vi "FPGA AIT 429 RT Driver VI.vi"(7 "Operation":T1, 11 "Device Reference in":T2 format="%.0x") -> (0 "Error Code":i32)   [LabVIEW 2012]
uses:
  <vilib>/NI Veristand/Custom Device API/Custom Device Item Ref.ctl
  <vilib>/NI Veristand/Custom Device API/Hardware Interface Driver VI Operation.ctl
  <vilib>/NI Veristand/Custom Device API/Custom Device Channel Type.ctl
  <vilib>/NI Veristand/Custom Device API/Data Reference.ctl
  SEA 9811 FPGA driver/RT/Typdefs/SEA9811_RT_data_cluster.ctl
  SEA 9811 FPGA driver/RT/Typdefs/FPGA ref.ctl
  SEA 9811 FPGA driver/RT/Typdefs/SEA9811_RT_conf_cluster.ctl
  <vilib>/userdefined/High Color/nirio_resource_hc.ctl
  SEA 9811 FPGA driver/FPGA/SEA-9811_ReceiverAndTransmitter/SubVIs/SEA-9811_ReceiverAndTransmitter_RCR.ctl
  SEA 9811 FPGA driver/FPGA/SEA-9811_ReceiverAndTransmitter/SubVIs/SEA-9811_ReceiverAndTransmitter_TCR.ctl
  <vilib>/NI Veristand/Custom Device API/Data Access Type.ctl
  <vilib>/NI Veristand/Custom Device API/Get Item Property (String).vi
  SEA 9811/Source/Shared/Constants.vi
  <vilib>/NI Veristand/Custom Device API/Global Data Refs.vi
  <vilib>/NI Veristand/Custom Device API/Custom Device API.lvlib
  SEA 9811/Source/Shared/SEA 9811 Shared.lvlib
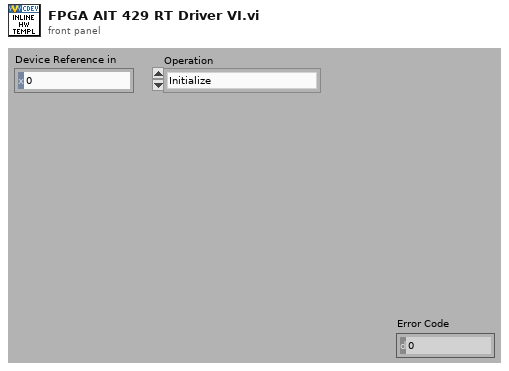
[diagram p1: front panel]
types:
  T1 = typedef "Custom Device API.lvlib/Hardware Interface Driver VI Operation.ctl" = enum16{"Initialize", "Start", "Read Data from HW", "Write Data to HW", "Close"}
  T2 = typedef "Custom Device API.lvlib/Custom Device Item Ref.ctl" = u64
  T3 = typedef "Custom Device API.lvlib/Data Reference.ctl" = i32
  T4 = typedef "SEA9811_RT_data_cluster.ctl" = cluster{"FPGA VI Reference":T5, "Incoming channels":dbl[], "words_timestamps":dbl[]}
  T5 = typedef "FPGA ref.ctl" = refnum<k20>
  T6 = cluster{"Input Values":dbl[], "Input Refs":T3[], "Output Values":dbl[], "Output Refs":T3[], "SEA9811_RT_data out":T4, "Device Error":errorcluster}
  T7 = typedef "SEA9811_RT_conf_cluster.ctl" = cluster{"FPGA resource name":T8, "Rx ch conf (0..7)":cluster{"Rx Channel Number (0..7)":u8, "Rx Label Filter":cluster{"Label 00":u8, "Label 01":u8, "Label 02":u8, "Label 03":u8, "Label 04":u8, "Label 05":u8, "Label 06":u8, "Label 07":u8, "Label 08":u8, "Label 09":u8, "Label 10":u8, "Label 11":u8, "Label 12":u8, "Label 13":u8, "Label 14":u8, "Label 15":u8}, "Receiver Control Register (RCR)":T9}[], "Transmitter Control Register (TCR)":T10}
  T8 = typedef "nirio_resource_hc.ctl" = tag
  T9 = typedef "SEA-9811_ReceiverAndTransmitter_RCR.ctl" = cluster{"RCR0: Data rate = ARINC 429 High-Speed (0) or Low-Speed (1)":bool, "RCR1: not used":bool, "RCR2: Label recognition for this channel enabled (1) or disabled (0)":bool, "RCR3: Receiver channel disabled (1) or enabled (0)":bool, "RCR4: Odd parity check for this channel enabled (1) or disabled (0":bool, "RCR5: Receiver normal operation (1) or loopback mode (0)":bool, "RCR6: Receiver Decoder disabled (0) or enabled (1) -> ARINC bits 10 and 9 must match RCR7 and RCR8":bool, "RCR7: If receiver decoder is enabled (RCR6=1), the ARINC bit 10 must match this bit":bool, "RCR8: If receiver decoder is enabled (RCR6=1), the ARINC bit 9 must match this bit":bool, "RCR9: Label bit order for this channel non-reversed (1) or reversed (0)":bool, "RCR10: not used":bool, "RCR11: not used":bool, "RCR12: not used":bool, "RCR13: not used":bool, "RCR14: not used":bool, "RCR15: not used":bool}
  T10 = typedef "SEA-9811_ReceiverAndTransmitter_TCR.ctl" = cluster{"TCR0: not used":bool, "TCR1: not used":bool, "TCR2: not used":bool, "TCR3: Transmitter Parity Bit Enable: 32nd bit is parity (1) or data (0)":bool, "TCR4: not used":bool, "TCR5: not used":bool, "TCR6: not used":bool, "TCR7: not used":bool, "TCR8: not used":bool, "TCR9: Transmitter Parity Select: odd parity (0) or even parity (1)":bool, "TCR10: Transmitter Data Rate: ARINC 429 high-speed (0) or low-speed (1)":bool, "TCR11: ARINC Label Bit Order: label bit order reversed (0) or not reversed (1)":bool, "TCR12: Disable Line Driver: normal operation (0) or transmitter disabled (1)":bool, "TCR13: Tansmit whenever data is available in FIFO (1) or only start by instruction \"Enable Transmission\" (0)":bool, "TCR14: not used":bool, "TCR15: not used":bool}
  T11 = typedef "Custom Device API.lvlib/Custom Device Channel Type.ctl" = enum16{"Input", "Output"}
  T12 = typedef "Custom Device API.lvlib/Data Access Type.ctl" = enum16{"Read", "Write"}
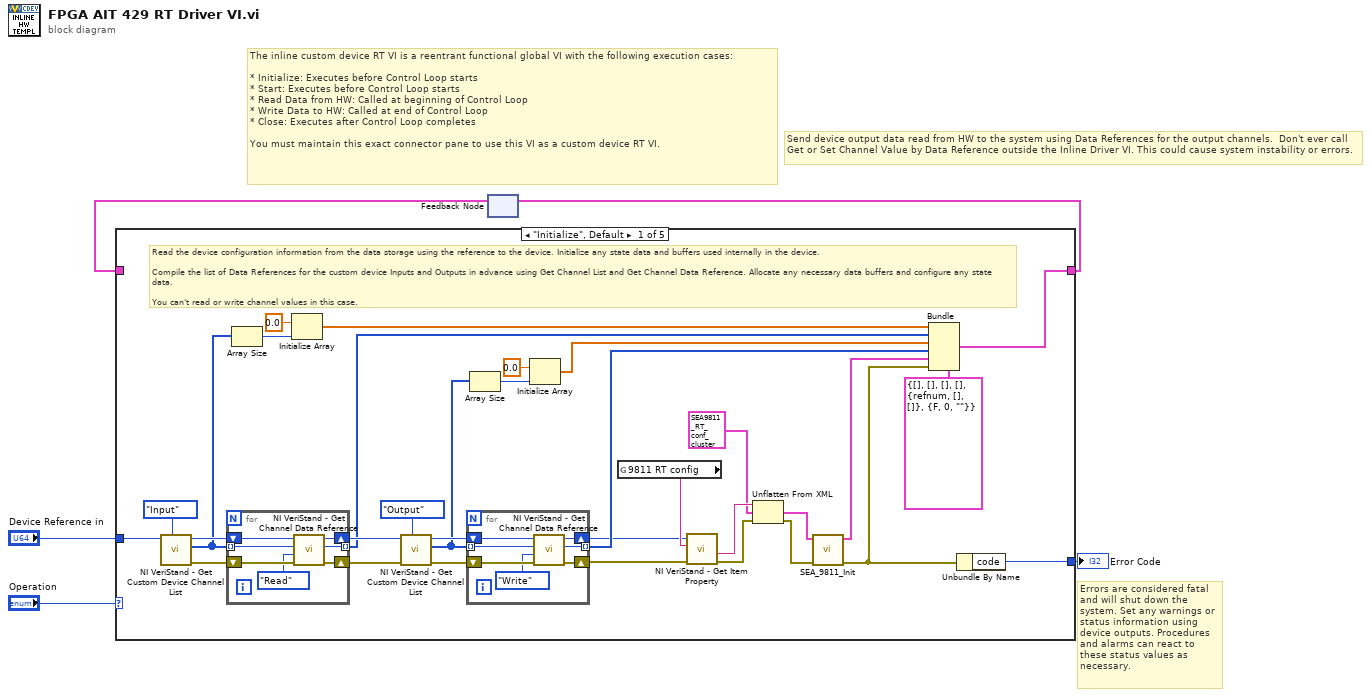
[diagram p0: block diagram]
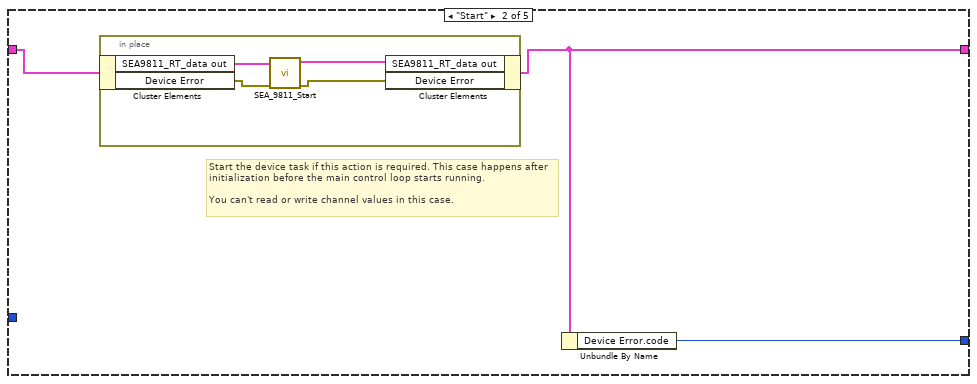
[diagram p2: hidden frame]
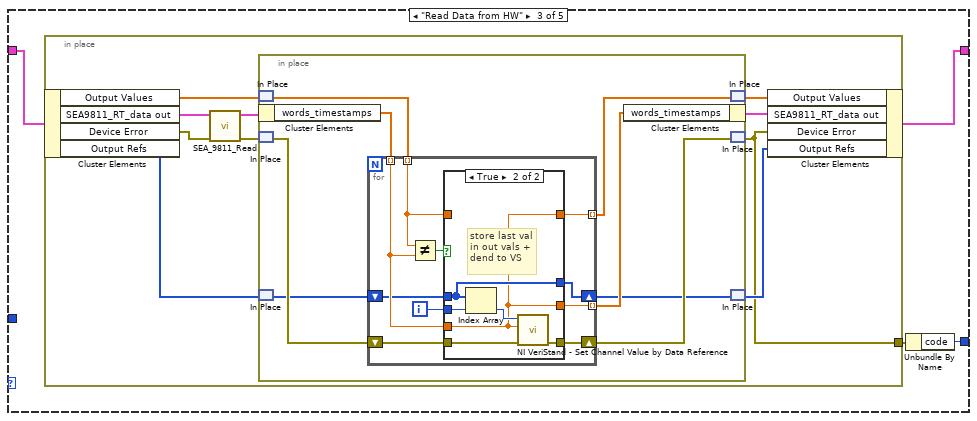
[diagram p3: hidden frame]
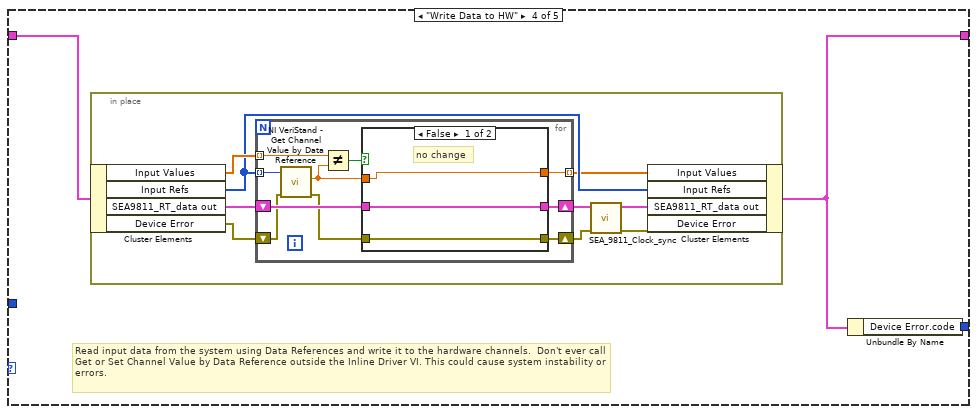
[diagram p5: hidden frame]
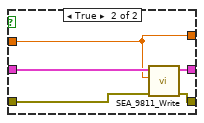
[diagram p6: hidden frame]
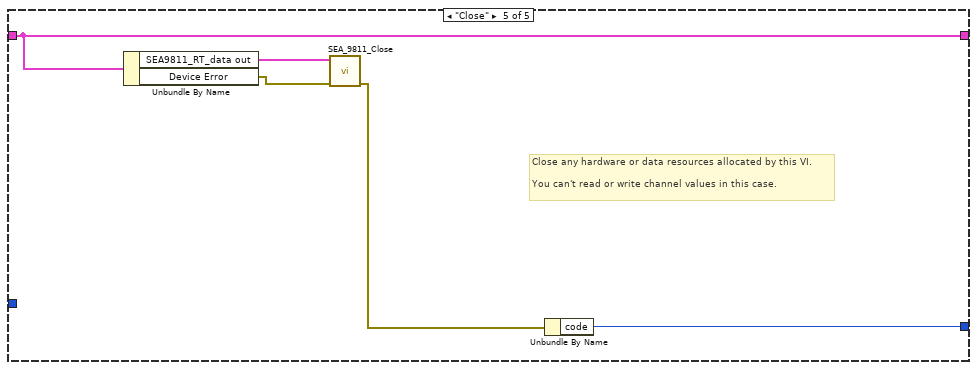
[diagram p7: hidden frame]
diagram:
  # "Send device output data read from HW to the system using Data References for the output channels.  Don't ever call Get or Set Channel Value by Data Reference outside the Inline Driver VI. This could cause system instability or errors."
  # "Errors are considered fatal and will shut down the system. Set any warnings or status information using device outputs. Procedures and alarms can react to these status values as necessary."
  # "The inline custom device RT VI is a reentrant functional global VI with the following execution cases:\n\n* Initialize: Executes before Control Loop starts\n* Start: Executes before Control Loop starts\n* Read Data from HW: Called at beginning of Control Loop\n* Write Data to HW: Called at end of Control Loop\n* Close: Executes after Control Loop completes\n\nYou must maintain this exact connector pane to use this VI as a custom device RT VI."
  n1 = feedback #1() -> (w3:T6)  [unwired: 1 out]
  n2 = case shown="\"Initialize\", Default" "Operation" {
    tunnel: [w32 w52 w60 w101 w131] -> w4
    tunnel: w3 -> [_ w53 w61 w102 w131]
    tunnel: "Device Reference in" -> [w33 _ _ _ _]
    tunnel: [w31 w54 w62 _ w134] -> w1
    frame "Initialize", Default {
      # "Read the device configuration information from the data storage using the reference to the device. Initialize any state data and buffers used internally in the device.\n\nCompile the list of Data References for the custom device Inputs and Outputs in advance using Get Channel List and Get Channel Data Reference. Allocate any necessary data buffers and configure any state data.\n\nYou can't read or write channel values in this case."
      n3 = call <vilib>:"NI VeriStand - Get Custom Device Channel List.vi"("Channel Type"=Custom_Device_Channel_Type."Input", "Device Ref in"=w33) -> ("error out"=w29:errorcluster, "Specified Channel Ref List"=w28:T2[], "Device Ref out"=w30:T2)  [unwired: 1 in, 6 out]
      n4 = for {
        shift-right: [w46] -> w24
        shift-left: w30 -> [w50]
        tunnel: w28 -> [w49] mode=indexing
        shift-right: [w47] -> w23
        shift-left: w29 -> [w51]
        tunnel: [w45] -> w22 mode=indexing
        n5 = call <vilib>:"NI VeriStand - Get Channel Data Reference.vi"("error in (no error)"=w51, "Access"=Data_Access_Type."Read", "Channel Ref in"=w49, "Device Ref in"=w50) -> ("error out"=w47:errorcluster, "Channel Data Reference"=w45:T3, "Device Ref out"=w46:T2)  [unwired: 5 out]
      }
      n6 = Array Size(array=w28) -> (size(s)=w36:i32)
      n7 = Initialize Array(0.0 ("element"), w36) -> (w37:dbl[])
      n8 = call <vilib>:"NI VeriStand - Get Custom Device Channel List.vi"("Channel Type"=Custom_Device_Channel_Type."Output", "error in (no error)"=w23, "Device Ref in"=w24) -> ("error out"=w27:errorcluster, "Specified Channel Ref List"=w19:T2[], "Device Ref out"=w26:T2)  [unwired: 6 out]
      n9 = for {
        tunnel: w19 -> [w42] mode=indexing
        shift-right: [w40] -> w8
        shift-left: w27 -> [w44]
        tunnel: [w39] -> w17 mode=indexing
        shift-right: [w38] -> w9
        shift-left: w26 -> [w43]
        n10 = call <vilib>:"NI VeriStand - Get Channel Data Reference.vi"("error in (no error)"=w44, "Access"=Data_Access_Type."Write", "Channel Ref in"=w42, "Device Ref in"=w43) -> ("error out"=w40:errorcluster, "Channel Data Reference"=w39:T3, "Device Ref out"=w38:T2)  [unwired: 5 out]
      }
      n11 = Array Size(array=w19) -> (size(s)=w20:i32)
      n12 = Initialize Array(0.0 ("element"), w20) -> (w18:dbl[])
      n13 = global read "Constants.vi" "9811 RT config"() -> (w13:string)
      n14 = call-poly <vilib>:"NI VeriStand - Get Item Property.vi"("error in (no error)"=w8, "Property Name"=w13, "Item Ref in"=w9) -> ("error out"=w11:errorcluster, "Value"=w12:string)  [unwired: 5 in, 2 out]
      n15 = Unflatten From XML(xml string=w12, type=T7 {"FPGA resource name"="RIO0", "Rx ch conf (0..7)"=[{"Rx Channel Number (0..7)"=0, "Rx Label Filter"={"Label 00"=0, "Label 01"=0, "Label 02"=0, "Label 03"=0, "Label 04"=0, "Label 05"=0, "Label 06"=0, "Label 07"=0, "Label 08"=0, "Label 09"=0, "Label 10"=0, "Label 11"=0, "Label 12"=0, "Label 13"=0, "Label 14"=0, "Label 15"=0}, "Receiver Control Register (RCR)"={"RCR0: Data rate = ARINC 429 High-Speed (0) or Low-Speed (1)"=FALSE, "RCR1: not used"=FALSE, "RCR2: Label recognition for this channel enabled (1) or disabled (0)"=FALSE, "RCR3: Receiver channel disabled (1) or enabled (0)"=FALSE, "RCR4: Odd parity check for this channel enabled (1) or disabled (0"=FALSE, "RCR5: Receiver normal operation (1) or loopback mode (0)"=TRUE, "RCR6: Receiver Decoder disabled (0) or enabled (1) -> ARINC bits 10 and 9 must match RCR7 and RCR8"=FALSE, "RCR7: If receiver decoder is enabled (RCR6=1), the ARINC bit 10 must match this bit"=FALSE, "RCR8: If receiver decoder is enabled (RCR6=1), the ARINC bit 9 must match this bit"=FALSE, "RCR9: Label bit order for this channel non-reversed (1) or reversed (0)"=FALSE, "RCR10: not used"=FALSE, "RCR11: not used"=FALSE, "RCR12: not used"=FALSE, "RCR13: not used"=FALSE, "RCR14: not used"=FALSE, "RCR15: not used"=FALSE}}], "Transmitter Control Register (TCR)"={"TCR0: not used"=FALSE, "TCR1: not used"=FALSE, "TCR2: not used"=FALSE, "TCR3: Transmitter Parity Bit Enable: 32nd bit is parity (1) or data (0)"=FALSE, "TCR4: not used"=FALSE, "TCR5: not used"=FALSE, "TCR6: not used"=FALSE, "TCR7: not used"=FALSE, "TCR8: not used"=FALSE, "TCR9: Transmitter Parity Select: odd parity (0) or even parity (1)"=FALSE, "TCR10: Transmitter Data Rate: ARINC 429 high-speed (0) or low-speed (1)"=FALSE, "TCR11: ARINC Label Bit Order: label bit order reversed (0) or not reversed (1)"=FALSE, "TCR12: Disable Line Driver: normal operation (0) or transmitter disabled (1)"=FALSE, "TCR13: Tansmit whenever data is available in FIFO (1) or only start by instruction \"Enable Transmission\" (0)"=TRUE, "TCR14: not used"=FALSE, "TCR15: not used"=FALSE}} ("SEA9811_conf_cluster 2"), error in (no error)=w11) -> (value=w6:T7, error out=w7:errorcluster)
      n16 = call "SEA_9811_Init.vi"("error in"=w7, "SEA9811_conf_cluster"=w6) -> ("error out"=w14:errorcluster, "SEA9811_RT_data out"=w15:T4)  [unwired: 8 in]
      n17 = Bundle(cluster=T6 {"Input Values"=[], "Input Refs"=[], "Output Values"=[], "Output Refs"=[], "SEA9811_RT_data out"={"FPGA VI Reference"=refnum, "Incoming channels"=[], "words_timestamps"=[]}, "Device Error"={"status"=FALSE, "code"=0, "source"=""}}, "Input Values"=w37, "Input Refs"=w22, "Output Values"=w18, "Output Refs"=w17, "SEA9811_RT_data out"=w15, "Device Error"=w14) -> (w32:T6)
      n18 = Unbundle By Name(w14) -> ("code"=w31:i32)
    }
    frame "Start" {
      # "Start the device task if this action is required. This case happens after initialization before the main control loop starts running.\n\nYou can't read or write channel values in this case."
      n19 = in-place {
        n20 = in-place-cluster #2(w53) -> ("SEA9811_RT_data out"=w58:T4, "Device Error"=w57:errorcluster)
        n21 = call "SEA_9811_Start.vi"("error in (no error)"=w57, "SEA9811_RT_data in"=w58) -> ("error out"=w55:errorcluster, "SEA9811_RT_data out"=w56:T4)  [unwired: 8 in]
        n22 = in-place-cluster #2("SEA9811_RT_data out"=w56, "Device Error"=w55) -> (w52:T6)
      }
      n23 = Unbundle By Name(w52) -> ("Device Error.code"=w54:i32)
    }
    frame "Read Data from HW" {
      n24 = in-place {
        in-place-border: [w64] -> w59
        n25 = in-place-cluster #3(w61) -> ("Output Values"=w69:dbl[], "SEA9811_RT_data out"=w71:T4, "Device Error"=w72:errorcluster, "Output Refs"=w67:T3[])
        n26 = call "SEA_9811_Read.vi"("error in (no error)"=w72, "SEA9811_RT_data in"=w71) -> ("error out"=w68:errorcluster, "SEA9811_RT_data out"=w70:T4)  [unwired: 6 in, 2 out]
        n27 = in-place {
          n28 = in-place-match #4(w69) -> (w79:dbl[])
          n29 = in-place-cluster #5(w70) -> ("words_timestamps"=w78:dbl[])
          n30 = in-place-match #6(w68) -> (w80:errorcluster)
          n31 = in-place-match #7(w67) -> (w77:T3[])
          n32 = for {
            tunnel: w79 -> [w84] mode=indexing
            tunnel: w78 -> [w89] mode=indexing
            shift-right: [w85] -> w74
            shift-left: w80 -> [w86]
            tunnel: [w83] -> w75 mode=indexing
            tunnel: [w82] -> w76 mode=indexing
            shift-right: [w81] -> w73
            shift-left: w77 -> [w88]
            i -> [w87]
            n33 = Not Equal?(x=w84, y=w89) -> (x != y?=w90:bool)
            n34 = case shown="True" w90 {
              tunnel: w89 -> [w91 w95]
              tunnel: w88 -> [w92 w96]
              tunnel: w87 -> [_ w100]
              tunnel: w86 -> [w94 w98]
              tunnel: [w94 w97] -> w85
              tunnel: w84 -> [w93 _]
              tunnel: [w93 w95] -> w83
              tunnel: [w91 w95] -> w82
              tunnel: [w92 w96] -> w81
              frame False {
              }
              frame True {
                # "store last val\nin out vals +\ndend to VS"
                n35 = Index Array(array=w96, index=w100) -> (element=w99:T3)
                n36 = call <vilib>:"NI VeriStand - Set Channel Value by Data Reference.vi"("error in (no error)"=w98, "Value"=w95, "Data Reference in"=w99) -> ("error out"=w97:errorcluster)  [unwired: 8 out]
              }
            }
          }
          n37 = in-place-cluster #5("words_timestamps"=w76) -> (w63:T4)
          n38 = in-place-match #4(w75) -> (w66:dbl[])
          n39 = in-place-match #6(w74) -> (w64:errorcluster)
          n40 = in-place-match #7(w73) -> (w65:T3[])
        }
        n41 = in-place-cluster #3("Output Values"=w66, "SEA9811_RT_data out"=w63, "Device Error"=w64, "Output Refs"=w65) -> (w60:T6)
      }
      n42 = Unbundle By Name(w59) -> ("code"=w62:i32)
    }
    frame "Write Data to HW" {
      # "Read input data from the system using Data References and write it to the hardware channels.  Don't ever call Get or Set Channel Value by Data Reference outside the Inline Driver VI. This could cause system instability or errors."
      n43 = in-place {
        n44 = in-place-cluster #8(w102) -> ("Input Values"=w105:dbl[], "Input Refs"=w104:T3[], "SEA9811_RT_data out"=w111:T4, "Device Error"=w110:errorcluster)
        n45 = for {
          shift-right: [w120] -> w109
          shift-left: w111 -> [w121]
          shift-right: [w119] -> w106
          shift-left: w110 -> [w117]
          tunnel: w104 -> [w118] mode=indexing
          tunnel: w105 -> [w116] mode=indexing
          tunnel: [w112] -> w103 mode=indexing
          n46 = call <vilib>:"NI VeriStand - Get Channel Value by Data Reference.vi"("error in (no error)"=w117, "Data Reference in"=w118) -> ("error out"=w114:errorcluster, "Value"=w113:dbl)  [unwired: 8 in]
          n47 = Not Equal?(x=w116, y=w113) -> (x != y?=w115:bool)
          n48 = case shown="False" w115 {
            tunnel: w121 -> [w124 w129]
            tunnel: [w124 w128] -> w120
            tunnel: [w123 w127] -> w119
            tunnel: w114 -> [w123 w126]
            tunnel: w113 -> [w122 w125]
            tunnel: [w122 w125] -> w112
            frame False {
              # "no change"
            }
            frame True {
              n49 = call "SEA_9811_Write.vi"("error in (no error)"=w126, "Tx Data"=w125, "SEA9811_RT_data in"=w129) -> ("error out"=w127:errorcluster, "SEA9811_RT_data out"=w128:T4)  [unwired: 7 in]
            }
          }
        }
        n50 = call "SEA_9811_Clock_sync.vi"("error in (no error)"=w106, "SEA9811_RT_data in"=w109) -> ("error out"=w107:errorcluster, "SEA9811_RT_data out"=w108:T4)  [unwired: 8 in]
        n51 = in-place-cluster #8("Input Values"=w103, "Input Refs"=w104, "SEA9811_RT_data out"=w108, "Device Error"=w107) -> (w101:T6)
      }
      n52 = Unbundle By Name(w101) -> ()  [unwired: 1 out]
    }
    frame "Close" {
      # "Close any hardware or data resources allocated by this VI.\n\nYou can't read or write channel values in this case."
      n53 = Unbundle By Name(w131) -> ("SEA9811_RT_data out"=w133:T4, "Device Error"=w132:errorcluster)
      n54 = call "SEA_9811_Close.vi"("error in (no error)"=w132, "SEA9811_RT_data in"=w133) -> ("error out"=w130:errorcluster)  [unwired: 9 in]
      n55 = Unbundle By Name(w130) -> ("code"=w134:i32)
    }
  }
  "Error Code" <- w1
  n56 = feedback-in #1(w4) -> ()
